vi "Write Channels to DAQ.vi"(8 "error in (no error)":errorcluster, 11 "Sequencer in":refnum<class "Sequencer.lvclass">) -> (0 "error out":errorcluster, 3 "Sequencer out":refnum<class "Sequencer.lvclass">)   [LabVIEW 2015, in "Sequencer.lvlib" / "Sequencer.lvclass"]
uses:
  Sequencer.lvclass
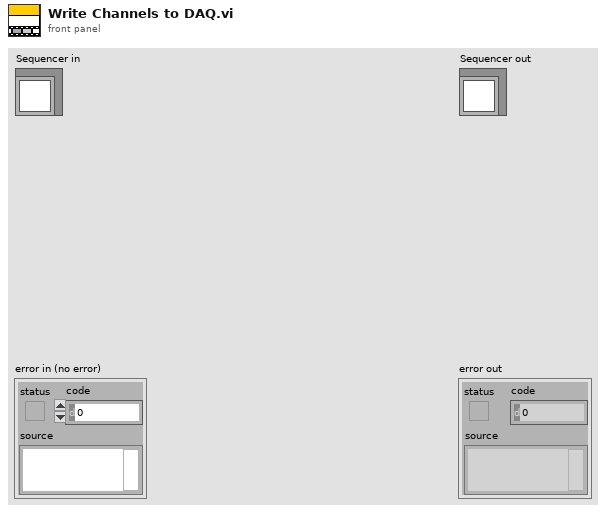
[diagram p1: front panel]
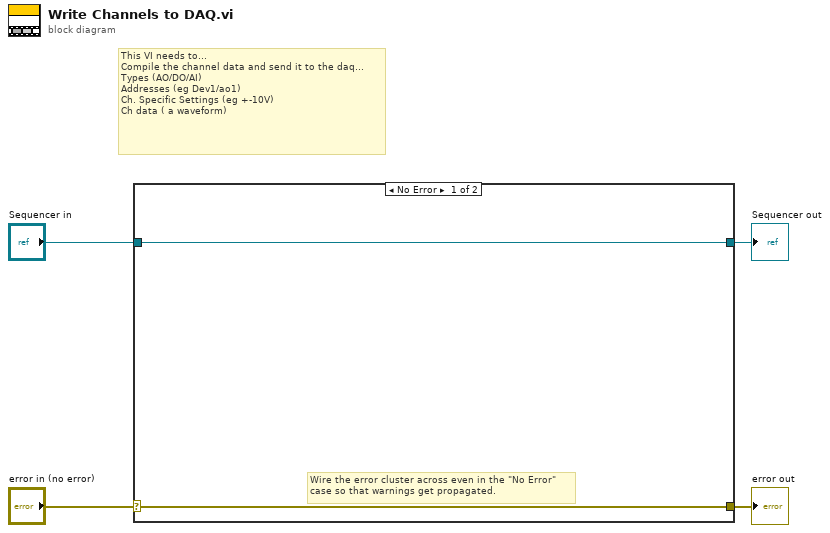
[diagram p0: block diagram]
diagram:
  # "This VI needs to...\nCompile the channel data and send it to the daq...\nTypes (AO/DO/AI)\nAddresses (eg Dev1/ao1)\nCh. Specific Settings (eg +-10V)\nCh data ( a waveform)"
  n1 = case shown="No Error" "error in (no error)" {
    selector: "error in (no error)" -> [w5 w8]
    tunnel: [w5 w8] -> w3
    tunnel: [w6 w7] -> w1
    tunnel: "Sequencer in" -> [w6 w7]
    frame No Error {
      # "Wire the error cluster across even in the \"No Error\"\ncase so that warnings get propagated."
    }
    frame Error {
    }
  }
  "error out" <- w3
  "Sequencer out" <- w1
